vi "CollectData.vi"(8 "error in (no error)":errorcluster, 11 "PTS-via-PB in":refnum<class "PTS-via-PB.lvclass">) -> (0 "error out":errorcluster, 3 "PTS-via-PB out":refnum<class "PTS-via-PB.lvclass">)   [LabVIEW 2013, in "PTS-via-PB.lvclass"]
uses:
  PTS-via-PB.lvclass
  Slave_Pulseblaster/Slave_Pulseblaster.lvclass
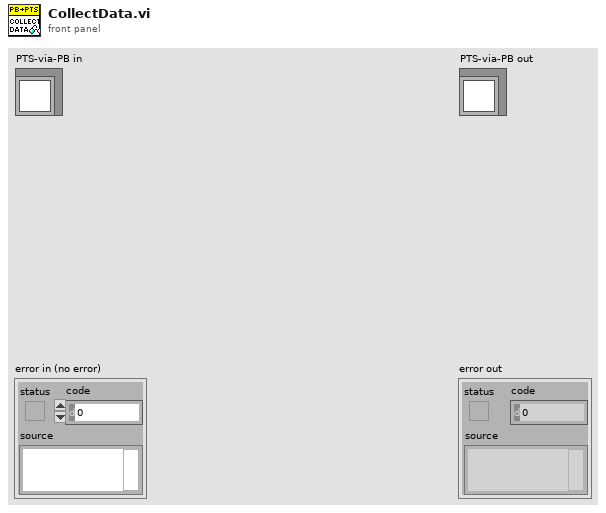
[diagram p1: front panel]
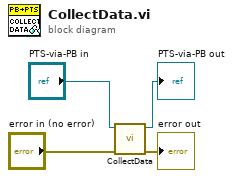
[diagram p0: block diagram]
diagram:
  n1 = call-parent "CollectData.vi"("error in (no error)"="error in (no error)", "Slave_Pulseblaster in"="PTS-via-PB in") -> ("error out"=→"error out":errorcluster, "Slave_Pulseblaster out"=→"PTS-via-PB out":refnum<class "PTS-via-PB.lvclass">)  [unwired: 8 in]
